vi "External Sensors.vi"(8 "error in (no error)":errorcluster, 11 "output cluster":T2) -> (0 "error out":errorcluster)   [LabVIEW 2016]
uses:
  Queue Cluster TD.ctl
  Queue Attributes TD.ctl
  Queue Enum TD.ctl
  External data TD.ctl
  <vilib>/DAQmx/read.llb/DAQmx Read (Analog 2D DBL NChan NSamp).vi
  <vilib>/DAQmx/miscellaneous.llb/DAQmx Fill In Error Info.vi
  <vilib>/Utility/file.llb/Write Delimited Spreadsheet (string).vi
panel:
  out "External Sensors":cluster{"[0]":dbl, "[1]":dbl, "[2]":dbl}[](graph)
  in  "samples per read":i32=100
  in  "External Data TD":T1
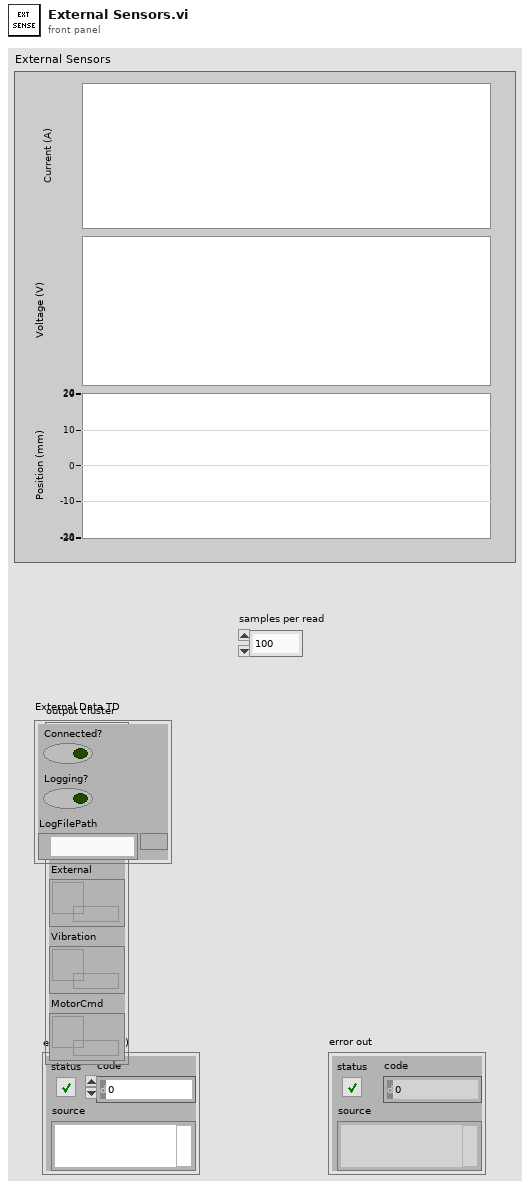
[diagram p1: front panel]
types:
  T1 = typedef "External Data TD.ctl" = cluster{"Connected?":bool, "Logging?":bool, "LogFilePath":path}
  T2 = typedef "Queue Cluster TD.ctl" = cluster{"Main":refnum<queue>, "Intrinsic":refnum<queue>, "External":refnum<queue>, "Vibration":refnum<queue>, "MotorCmd":refnum<queue>}
  T3 = typedef "Queue Attributes TD.ctl" = cluster{"State":T4, "String":string, "Boolean":bool, "Double":dbl, "U16":u16}
  T4 = typedef "Queue Enum TD.ctl" = enum16{"Stop", "Start", "Update D_HW", "Initialize", "Exit", "Read", "Write", "Plot", "Log", "Stop Log", "Start Log", "Wait"}
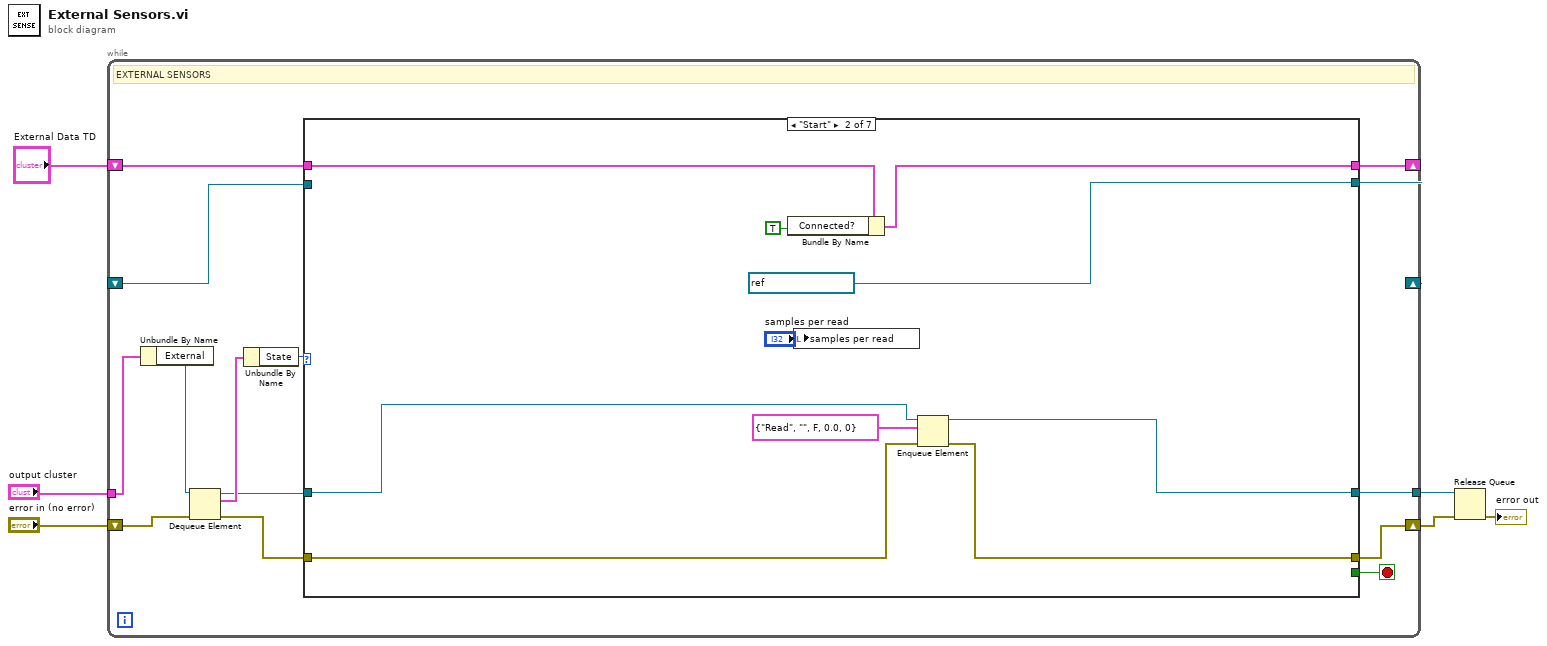
[diagram p0: block diagram]
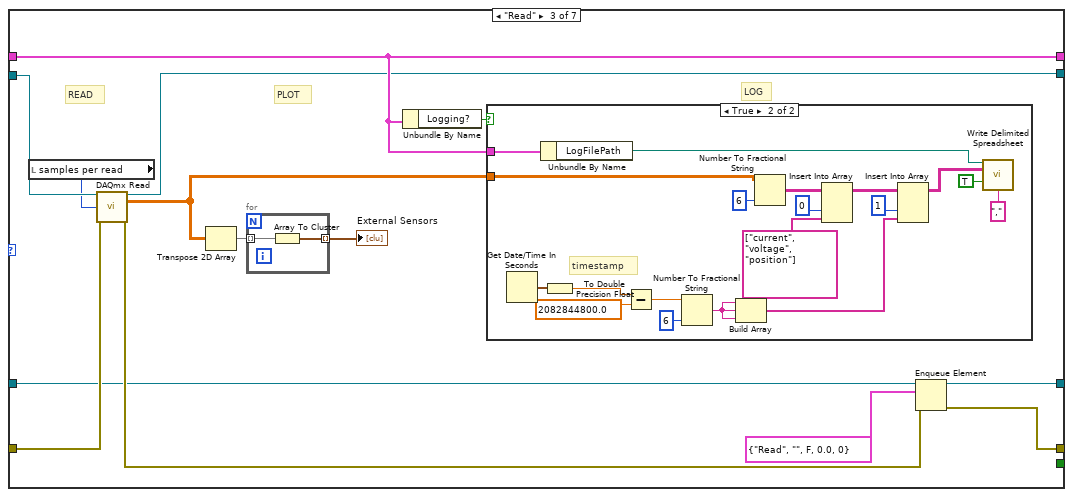
[diagram p3: hidden frame]
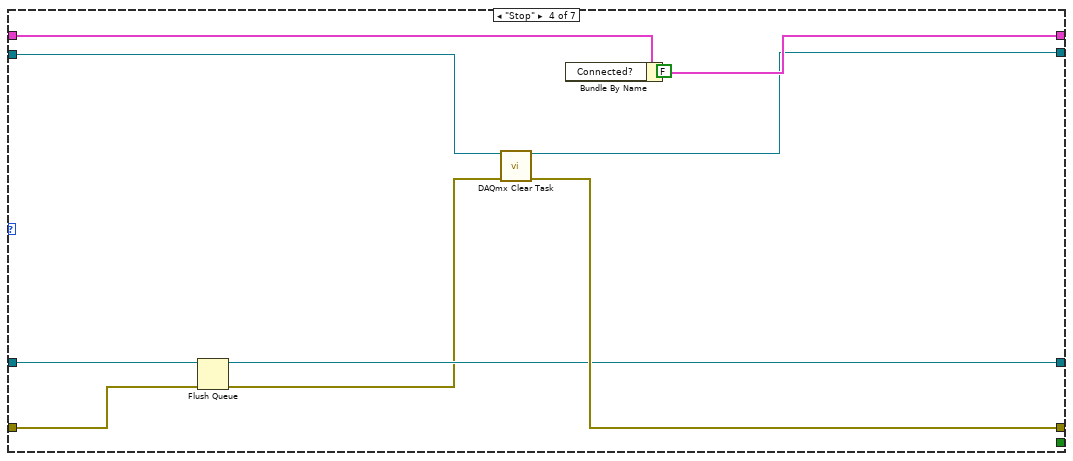
[diagram p5: hidden frame]
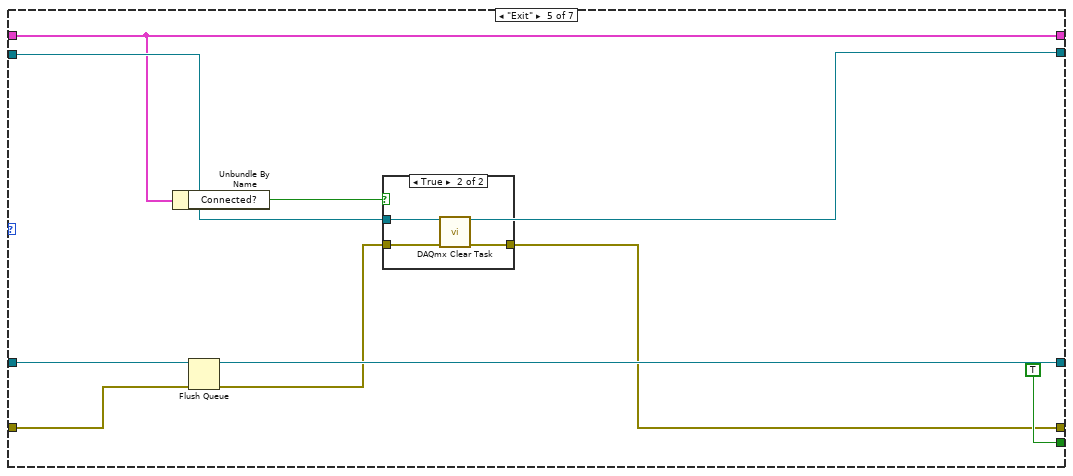
[diagram p6: hidden frame]
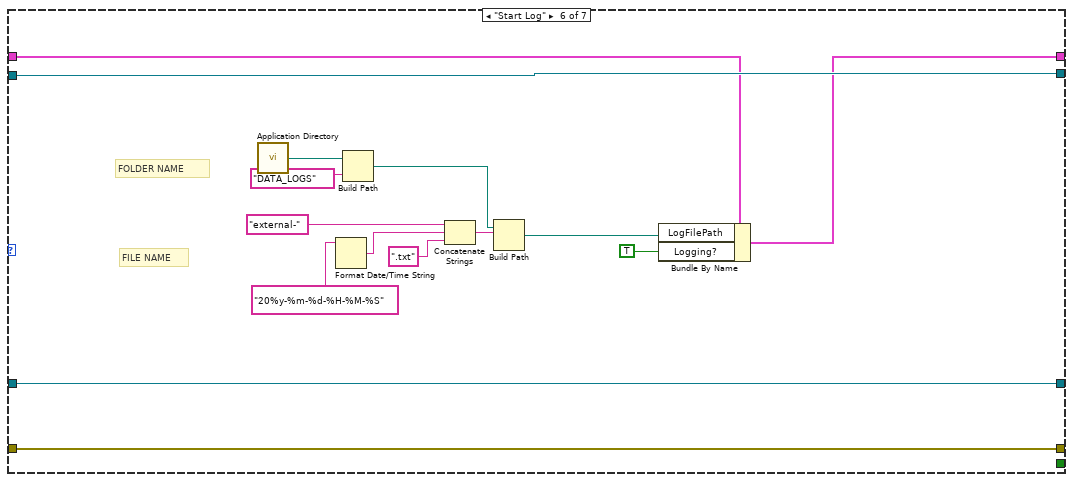
[diagram p8: hidden frame]
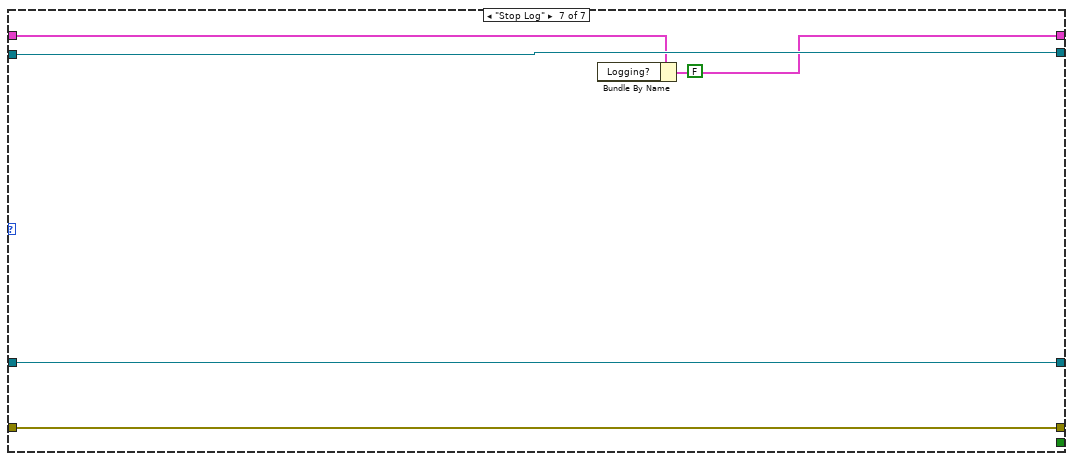
[diagram p9: hidden frame]
diagram:
  n1 = while {
    tunnel: "output cluster" -> [w7]
    tunnel: [w15] -> w5
    shift-right: [w14] -> w6
    shift-left: "error in (no error)" -> [w19]
    shift-right: [w11] -> _
    shift-left: _ -> [w10]
    shift-right: [w8] -> _
    shift-left: "External Data TD" -> [w9]
    stop <- w12 stop-if-true
    # "EXTERNAL SENSORS"
    n2 = Unbundle By Name(w7) -> ("External"=w20:refnum<queue>)
    n3 = Dequeue Element(queue=w20, error in (no error)=w19) -> (queue out=w16:refnum<queue>, element=w18:T3, error out=w17:errorcluster)  [unwired: 1 in, 1 out]
    n4 = Unbundle By Name(w18) -> ("State"=w13:T4)
    n5 = case shown="\"Start\"" w13 {
      tunnel: w17 -> [w21 w26 w45 w74 w81 w92 w107]
      tunnel: w16 -> [w22 w33 w41 w73 w83 w106 w112]
      tunnel: [w22 w32 w47 w72 w82 w106 w112] -> w15
      tunnel: [w21 w34 w48 w75 w79 w92 w107] -> w14
      tunnel: [_ _ _ _ TRUE _ _] -> w12
      tunnel: [w24 refnum<k21> "ExternalTask" ("DAQmx Task Name") w35 w70 w86 w105 w111] -> w11
      tunnel: w10 -> [w24 _ w43 w70 w86 w105 w111]
      tunnel: w9 -> [w23 w31 w39 w78 w85 w104 w110]
      tunnel: [w23 w30 w39 w77 w85 w103 w109] -> w8
      frame "Initialize", Default {
      }
      frame "Start" {
        n6 = Bundle By Name(cluster=w31, "Connected?"=TRUE) -> (w30:T1)
        n7 = local write "samples per read"("samples per read") -> ()
        n8 = Enqueue Element(queue=w33, element=T3 {"State"=enum."Read", "String"="", "Boolean"=FALSE, "Double"=0.0, "U16"=0}, error in (no error)=w26) -> (queue out=w32:refnum<queue>, error out=w34:errorcluster)  [unwired: 1 in, 1 out]
      }
      frame "Read" {
        # "LOG"
        # "PLOT"
        # "READ"
        n9 = local read "samples per read"() -> (w42:i32)
        n10 = call-poly <vilib>:"DAQmx Read.vi"("task/channels in"=w43, "number of samples per channel"=w42, "error in"=w45) -> ("task out"=w35:refnum<k21>, "data"=w38:dbl[][], "error out"=w44:errorcluster)  [unwired: 10 in]
        n11 = Transpose 2D Array(2D array=w38) -> (transposed array=w37:dbl[][])
        n12 = for {
          tunnel: w37 -> [w69] mode=indexing
          tunnel: [w68] -> w36 mode=indexing
          n13 = Array To Cluster(array=w69) -> (cluster=w68:cluster{"[0]":dbl, "[1]":dbl, "[2]":dbl})
        }
        "External Sensors" <- w36
        n14 = Unbundle By Name(w39) -> ("Logging?"=w40:bool)
        n15 = case shown="True" w40 {
          tunnel: w39 -> [_ w55]
          tunnel: w38 -> [_ w51]
          frame False {
          }
          frame True {
            # "timestamp"
            n16 = Get Date/Time In Seconds() -> (seconds since 1Jan1904=w65:timestamp)
            n17 = Unbundle By Name(w55) -> ("LogFilePath"=w54:path)
            n18 = To Double Precision Float(number=w65) -> (double precision float=w66:dbl)
            n19 = Subtract(x=w66, y=2082844800.0 ("Epoch Delta (s)")) -> (x-y=w53:dbl)
            n20 = Number To Fractional String(number=w53, precision (6)=i16 6) -> (F-format string=w59:string)  [unwired: 2 in]
            n21 = Build Array(w59, w59, w59) -> (w56:string[])
            n22 = Number To Fractional String(number=w51, precision (6)=i16 6) -> (F-format string=w50:string[][])  [unwired: 2 in]
            n23 = Insert Into Array(array=w50, index (col)=0 ("index (row)"), new element=string[] ["current", "voltage", "position"]) -> (w58:string[][])  [unwired: 1 in]
            n24 = Insert Into Array(array=w58, index (col)=1 ("index (row)"), new element=w56) -> (w49:string[][])  [unwired: 1 in]
            n25 = call-poly <vilib>:"Write Delimited Spreadsheet.vi"("file path (dialog if empty)"=w54, "2D data"=w49, "append to file? (new file:F)"=TRUE, "delimiter (\\t)"="," ("delimiter (\\t)")) -> ()  [unwired: 10 in, 2 out]
          }
        }
        n26 = Enqueue Element(queue=w41, element=T3 {"State"=enum."Read", "String"="", "Boolean"=FALSE, "Double"=0.0, "U16"=0}, error in (no error)=w44) -> (queue out=w47:refnum<queue>, error out=w48:errorcluster)  [unwired: 1 in, 1 out]
      }
      frame "Stop" {
        n27 = Flush Queue(queue=w73, error in (no error)=w74) -> (queue out=w72:refnum<queue>, error out=w71:errorcluster)  [unwired: 1 out]
        n28 = call <vilib>:"DAQmx Clear Task.vi"("task in"=w70, "error in"=w71) -> ("error out"=w75:errorcluster)  [unwired: 13 in]
        n29 = Bundle By Name(cluster=w78, "Connected?"=FALSE) -> (w77:T1)
      }
      frame "Exit" {
        n30 = Unbundle By Name(w85) -> ("Connected?"=w84:bool)
        n31 = Flush Queue(queue=w83, error in (no error)=w81) -> (queue out=w82:refnum<queue>, error out=w80:errorcluster)  [unwired: 1 out]
        n32 = case shown="True" w84 {
          tunnel: w86 -> [_ w91]
          tunnel: w80 -> [w88 w90]
          tunnel: [w88 w89] -> w79
          frame False {
          }
          frame True {
            n33 = call <vilib>:"DAQmx Clear Task.vi"("task in"=w91, "error in"=w90) -> ("error out"=w89:errorcluster)  [unwired: 13 in]
          }
        }
      }
      frame "Start Log" {
        # "FILE NAME"
        # "FOLDER NAME"
        n34 = call <vilib>:"Application Directory.vi"() -> ("Application Directory"=w97:path)
        n35 = Format Date/Time String(time format string (%c)="20%y-%m-%d-%H-%M-%S") -> (date/time string=w99:string)  [unwired: 2 in]
        n36 = Build Path(base path=w97, name or relative path="DATA_LOGS") -> (appended path=w98:path)
        n37 = Concatenate Strings("external-" ("string"), w99, ".txt") -> (w102:string)
        n38 = Build Path(base path=w98, name or relative path=w102) -> (appended path=w94:path)
        n39 = Bundle By Name(cluster=w104, "LogFilePath"=w94, "Logging?"=TRUE) -> (w103:T1)
      }
      frame "Stop Log" {
        n40 = Bundle By Name(cluster=w110, "Logging?"=FALSE) -> (w109:T1)
      }
    }
  }
  n41 = Release Queue(queue=w5, error in (no error)=w6) -> (error out=→"error out":errorcluster)  [unwired: 1 in, 2 out]
